vi "Data.vi"() -> ()   [LabVIEW 2018]
panel:
  out "运行参数":T1
  in  "电机":T2
  in  "能量计":T2
  in  "功率计":T2
  in  "偏振仪":T2
  in  "相机":T2
  in  "光谱仪":T2
  in  "示波器":T3={"Channel (0:Channel 1)"=enum."Channel 1", "电压范围"=0, "触发电压"=0, "时间范围"=0, " 示波器VISA"="TCPIP::192.168.129.100::INSTR"}
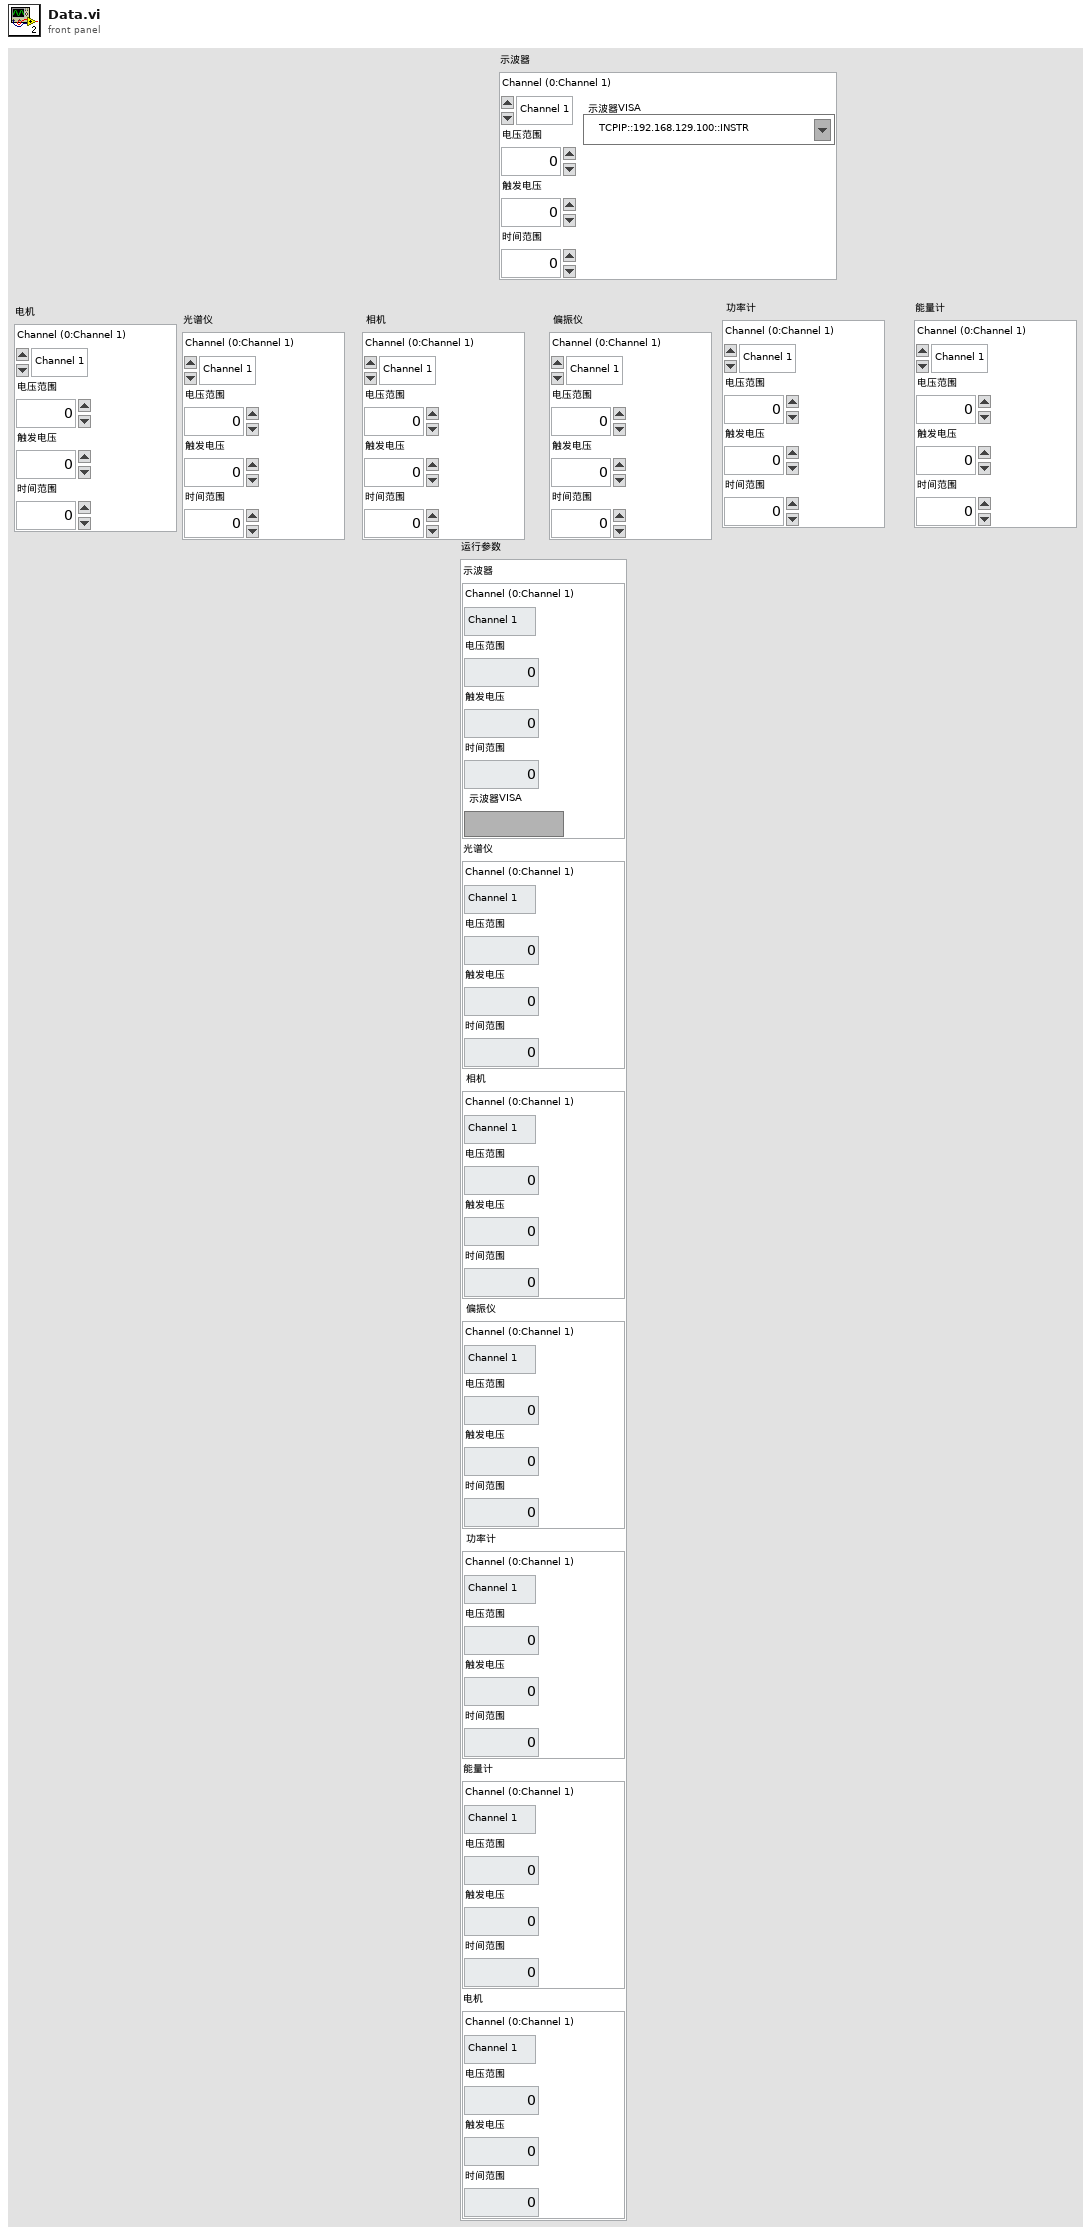
[diagram p1: front panel]
types:
  T1 = cluster{"示波器":cluster{"Channel (0:Channel 1)":enum16{"Channel 1", "Channel 2", "Channel 3", "Channel 4"}, "电压范围":u64, "触发电压":u64, "时间范围":u64, " 示波器VISA":refnum<visa-resource-name>}, "光谱仪":cluster{"Channel (0:Channel 1)":enum16{"Channel 1", "Channel 2", "Channel 3", "Channel 4"}, "电压范围":u64, "触发电压":u64, "时间范围":u64}, " 相机":cluster{"Channel (0:Channel 1)":enum16{"Channel 1", "Channel 2", "Channel 3", "Channel 4"}, "电压范围":u64, "触发电压":u64, "时间范围":u64}, " 偏振仪":cluster{"Channel (0:Channel 1)":enum16{"Channel 1", "Channel 2", "Channel 3", "Channel 4"}, "电压范围":u64, "触发电压":u64, "时间范围":u64}, " 功率计":cluster{"Channel (0:Channel 1)":enum16{"Channel 1", "Channel 2", "Channel 3", "Channel 4"}, "电压范围":u64, "触发电压":u64, "时间范围":u64}, "能量计":cluster{"Channel (0:Channel 1)":enum16{"Channel 1", "Channel 2", "Channel 3", "Channel 4"}, "电压范围":u64, "触发电压":u64, "时间范围":u64}, "电机":cluster{"Channel (0:Channel 1)":enum16{"Channel 1", "Channel 2", "Channel 3", "Channel 4"}, "电压范围":u64, "触发电压":u64, "时间范围":u64}}
  T2 = cluster{"Channel (0:Channel 1)":enum16{"Channel 1", "Channel 2", "Channel 3", "Channel 4"}, "电压范围":u64, "触发电压":u64, "时间范围":u64}
  T3 = cluster{"Channel (0:Channel 1)":enum16{"Channel 1", "Channel 2", "Channel 3", "Channel 4"}, "电压范围":u64, "触发电压":u64, "时间范围":u64, " 示波器VISA":refnum<visa-resource-name>}
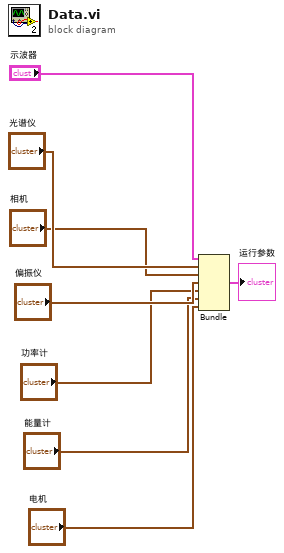
[diagram p0: block diagram]
diagram:
  n1 = Bundle("示波器"="示波器", "光谱仪"="光谱仪", "相机"="相机", "偏振仪"="偏振仪", "功率计"="功率计", "能量计"="能量计", "电机"="电机") -> (→"运行参数":T1)  [unwired: 1 in]
